vi "Q to wRL.vi"(2 "Wavelength":dbl format="%.5f", 3 "Q":cdb format="%.5f") -> (0 "Radius of Curvature":dbl format="%.2f", 1 "beam radius(w)":dbl format="%.2f")   [LabVIEW 2016]
panel:
  out "1/Q":cdb format="%.8f"
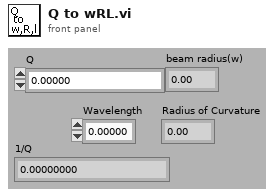
[diagram p1: front panel]
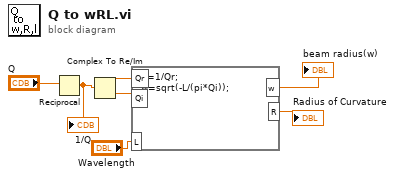
[diagram p0: block diagram]
diagram:
  n1 = Reciprocal(x="Q") -> (1/x=w5:cdb)
  "1/Q" <- w5
  n2 = Complex To Re/Im(x + iy=w5) -> (x=w2:dbl, y=w1:dbl)
  n3 = formula code="R=1/Qr;\nw=sqrt(-L/(pi*Qi));"("Qr"=w2, "Qi"=w1, "L"="Wavelength") -> ("w"=→"beam radius(w)":dbl, "R"=→"Radius of Curvature":dbl)
